vi "SRS 830 Get Data.vi"(2 "Point #":i32, 3 "Command String":string, 4 "Instrument Address":refnum<visa-resource-name>) -> (0 "Stop":bool, 1 "SRS 830 Output":dbl[](array[numeric]) format="%.2e")   [LabVIEW 2024]
doc: "This VI reads two channels of the PAR 5210 lockin. It will not work for the 5208. The output is an array of values. The input is the numeric GPIB address.\nScott Hannahs, F. Bitter National Magnet Lab, May 1993"
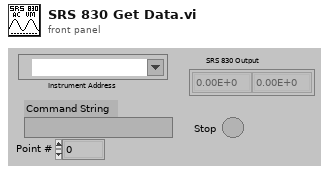
[diagram p1: front panel]
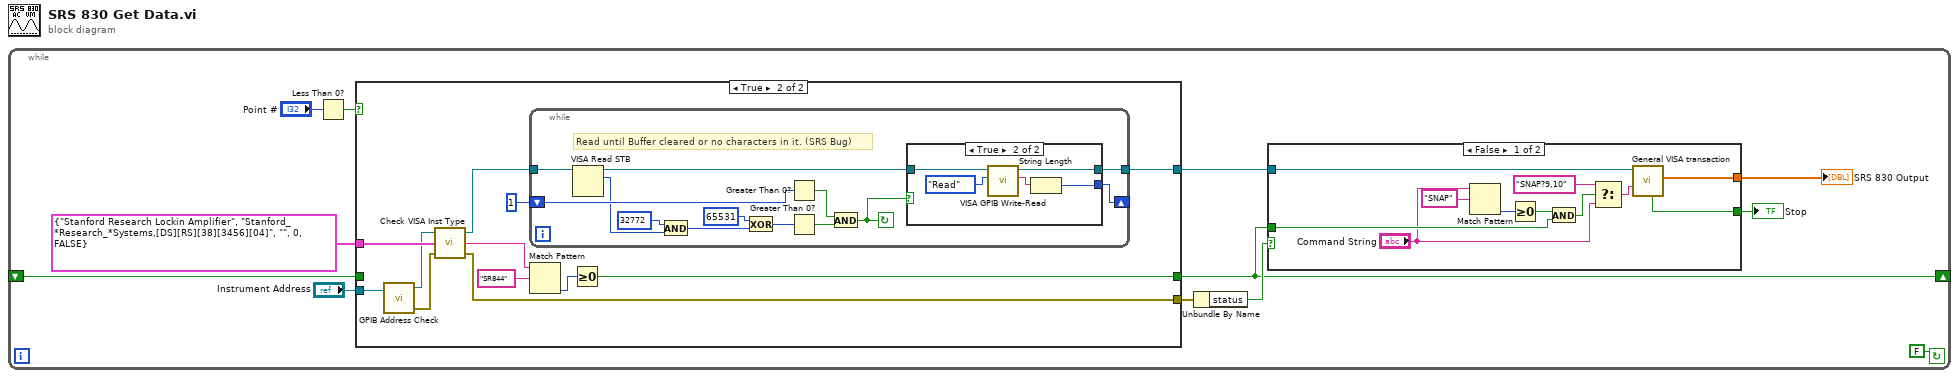
[diagram p0: block diagram]
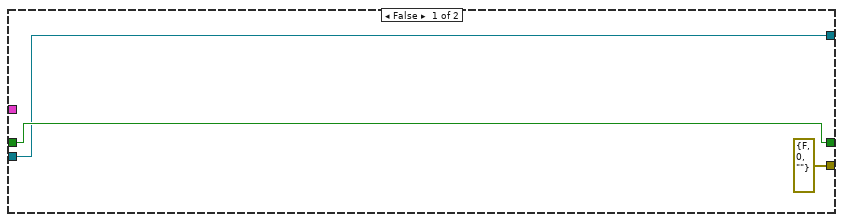
[diagram p2: hidden frame]
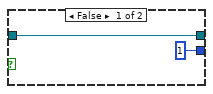
[diagram p3: hidden frame]
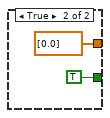
[diagram p4: hidden frame]
diagram:
  n1 = while {
    shift-left: _ -> [w4]
    shift-right: [w3] -> _
    stop <- FALSE continue-if-true
    n2 = Less Than 0?(x="Point #") -> (x < 0?=w9:bool)
    n3 = case shown="True" w9 {
      tunnel: "Instrument Address" -> [w13 w18]
      tunnel: [errorcluster {"status"=FALSE, "code"=0, "source"=""} ("error out") w19] -> w11
      tunnel: cluster{string, string, string, u32, bool} {"Stanford Research Lockin Amplifier", "Stanford_*Research_*Systems,[DS][RS][38][3456][04]", "", 0, FALSE} -> [_ w22]
      tunnel: [w14 w24] -> w3
      tunnel: w4 -> [w14 _]
      tunnel: [w13 w16] -> w1
      frame False {
      }
      frame True {
        n4 = call "GPIB Address Check.vi"("Instrument Address"=w18) -> ("dup VISA session"=w21:refnum<visa-resource-name>, "error out"=w23:errorcluster)  [unwired: 1 in, 1 out]
        n5 = call "Check VISA Inst Type.vi"("Error In"=w23, "Check Parameters"=w22, "VISA session"=w21) -> ("Error Out"=w19:errorcluster, "ID"=w20:string, "dup VISA session"=w17:refnum<visa-resource-name>)
        n6 = while {
          tunnel: w17 -> [w33]
          shift-left: 1 -> [w39]
          shift-right: [w37] -> _
          tunnel: [w28] -> w16
          stop <- w38 continue-if-true
          # "Read until Buffer cleared or no characters in it. (SRS Bug)"
          n7 = VISA Read STB(11:w33) -> (2:w31:u16, 3:w32:refnum<visa-resource-name>)  [unwired: 1 in, 1 out]
          n8 = And(x=u16 32772, y=w31) -> (x .and. y?=w34:u16)
          n9 = Exclusive Or(1:w34, 2:u16 65531) -> (0:w29:u16)
          n10 = Greater Than 0?(x=w39) -> (x > 0?=w40:bool)
          n11 = Greater Than 0?(x=w29) -> (x > 0?=w30:bool)
          n12 = And(x=w40, y=w30) -> (x .and. y?=w38:bool)
          n13 = case shown="True" w38 {
            tunnel: w32 -> [w41 w44]
            tunnel: [1 w47] -> w37
            tunnel: [w41 w43] -> w28
            frame False {
            }
            frame True {
              n14 = call "VISA GPIB Write-Read.vi"("Action"=enum16{"Write", "Read", "Write & Read"}."Read", "VISA resource name"=w44) -> ("String Returned"=w46:string, "dup VISA Session"=w43:refnum<visa-resource-name>)  [unwired: 6 in, 2 out]
              n15 = String Length(string=w46) -> (length=w47:i32)
            }
          }
        }
        n16 = Match Pattern(string=w20, regular expression="SR844") -> (offset past match=w25:i32)  [unwired: 1 in, 3 out]
        n17 = Greater Or Equal To 0?(x=w25) -> (x >= 0?=w24:bool)
      }
    }
    n18 = Unbundle By Name(w11) -> ("status"=w12:bool)
    n19 = case shown="False" w12 {
      tunnel: w1 -> [w48 _]
      tunnel: [w51 dbl[] [0.0]] -> w8
      tunnel: [w50 TRUE ("Stop")] -> w7
      tunnel: w3 -> [w55 _]
      frame False {
        n20 = Match Pattern(string="Command String", regular expression="SNAP") -> (offset past match=w57:i32)  [unwired: 1 in, 3 out]
        n21 = Greater Or Equal To 0?(x=w57) -> (x >= 0?=w56:bool)
        n22 = And(x=w56, y=w55) -> (x .and. y?=w54:bool)
        n23 = Select(t="SNAP?9,10", s=w54, f="Command String") -> (s? t:f=w49:string)
        n24 = call "General VISA transaction.vi"("Command String"=w49, "VISA Session"=w48) -> ("Measurement"=w51:dbl[], "Stop"=w50:bool)  [unwired: 4 in, 4 out]
      }
      frame True {
      }
    }
    "SRS 830 Output" <- w8
    "Stop" <- w7
  }
